vi "GetColoredBrush.vi"(0 "reference in":refnum<class "LcPictureBox.lvclass">, 1 "Alpha(100%)":dbl=100.0, 2 "Color(Black)":u32(colorbox), 3 "Pen(Width=1, Solid)":T1, 5 "Error In":errorcluster) -> (14 "reference out":refnum<class "LcPictureBox.lvclass">, 15 "SolidBrushRef":refnum<k24>, 19 "Error Out":errorcluster)   [LabVIEW 2020, in "LcPictureBox.lvclass"]
uses:
  LcPictureBox.lvclass
  Pen.ctl
  System.Drawing
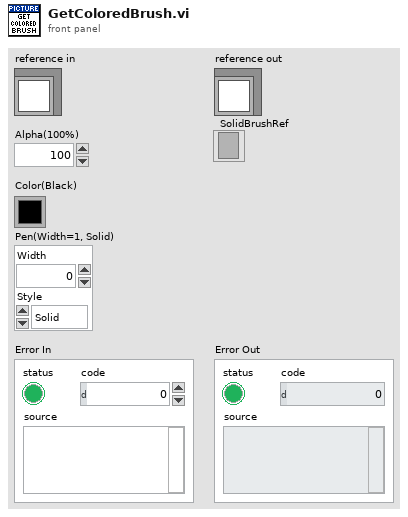
[diagram p1: front panel]
types:
  T1 = typedef "LcPictureBox.lvclass/Pen.ctl" = cluster{"Width":u16, "Style":enum32{"Solid", "Dash", "Dot", "DashDot", "DashDotDot"}}
  T2 = typedef "LcPictureBox.lvclass/ObjectAttributes.ctl" = cluster{"PictureBox":refnum<k24>, "ImageSize":cluster{"Width":i32, "Height":i32}, "PenMemory":map{cluster{"Alpha(100%)":dbl, "Color(Black)":u32, "Pen(Width=1, Solid)":T1}, refnum<k24>}, "GraphicsRef":refnum<k24>, "BrushMemory":map{cluster{"Alpha(100%)":dbl, "Color(Black)":u32}, refnum<k24>}, "Images":refnum<k24>[], "ImageIndex":i32, "BgColor(None)":u32, "LoadedImages":map{string, cluster{"ImageOut":refnum<k24>, "ImageSize":cluster{"Width":i32, "Height":i32}}}, "ColorsMemory":map{cluster{"Alpha(100%)":dbl, "Color(Black)":u32}, refnum<k24>}, "CacheSize":i32, "PictureBoxActiveXReference":refnum<vi>, "Scale":sgl, "Offset":cluster{"x":sgl, "y":sgl}, "zoom_center":cluster{"X":i32, "Y":i32}, "ImagesCreated":refnum<k24>[]}
  T3 = map{cluster{"Alpha(100%)":dbl, "Color(Black)":u32}, refnum<k24>}
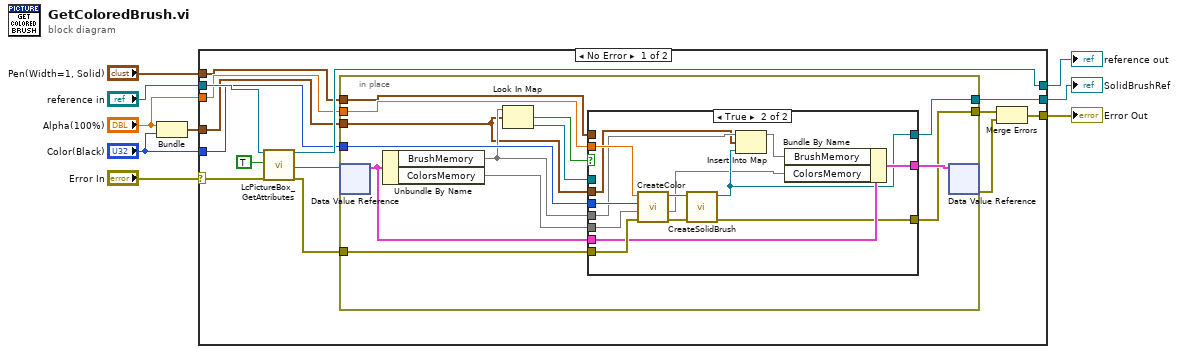
[diagram p0: block diagram]
diagram:
  n1 = Bundle("Alpha(100%)"="Alpha(100%)", "Color(Black)"="Color(Black)") -> (w5:cluster{"Alpha(100%)":dbl, "Color(Black)":u32})  [unwired: 1 in]
  n2 = case shown="No Error" "Error In" {
    selector: "Error In" -> [w22 w55]
    tunnel: [w19 w55] -> w8
    tunnel: [w20 w54] -> w6
    tunnel: "reference in" -> [w23 w54]
    tunnel: w5 -> [w16 _]
    tunnel: [w15 _] -> w4
    tunnel: "Alpha(100%)" -> [w14 _]
    tunnel: "Color(Black)" -> [w13 _]
    tunnel: "Pen(Width=1, Solid)" -> [w12 _]
    frame No Error {
      n3 = call "LcPictureBox_GetAttributes.vi"("reference in"=w23, "OnlyGetDvrReference(False)"=TRUE, "error in (no error)"=w22) -> ("reference out"=w20:refnum<class "LcPictureBox.lvclass">, "DataRef"=w18:refnum<data-value>, "error out"=w11:errorcluster)  [unwired: 13 in, 1 out]
      n4 = in-place {
        in-place-border: w16 -> [w25]
        in-place-border: [w32] -> w15
        in-place-border: w14 -> [w31]
        in-place-border: w13 -> [w30]
        in-place-border: w11 -> [w29]
        in-place-border: w12 -> [w28]
        in-place-border: [w27] -> w10
        n5 = in-place-dvr #1(w18) -> (w35:T2)  [unwired: 1 out]
        n6 = Unbundle By Name(w35) -> ("BrushMemory"=w26:T3, "ColorsMemory"=w24:T3)
        n7 = Look In Map(map=w26, key=w25) -> (key not found?=w34:bool, value=w33:refnum<k24>)  [unwired: 1 in]
        n8 = case shown="True" w34 {
          tunnel: [w37 w53] -> w36
          tunnel: w35 -> [w37 w48]
          tunnel: w33 -> [w39 _]
          tunnel: [w39 w43] -> w32
          tunnel: w31 -> [_ w52]
          tunnel: w30 -> [_ w51]
          tunnel: w29 -> [w38 w50]
          tunnel: w28 -> [_ _]
          tunnel: [w38 w40] -> w27
          tunnel: w26 -> [_ w47]
          tunnel: w25 -> [_ w45]
          tunnel: w24 -> [_ w42]
          frame False {
          }
          frame True {
            n9 = call "CreateColor.vi"("error in (no error)"=w50, "ColorsIn"=w42, "Color(Black)"=w51, "Alpha(100%)"=w52) -> ("error out"=w49:errorcluster, "ColorsOut"=w41:T3, "ColorRef"=w44:refnum<k24>)  [unwired: 5 in]
            n10 = call "CreateSolidBrush.vi"("error in (no error)"=w49, "ColorRef"=w44) -> ("error out"=w40:errorcluster, "SolidBrushRef"=w43:refnum<k24>)  [unwired: 8 in]
            n11 = Insert Into Map(map in=w47, key=w45, value=w43) -> (map out=w46:T3)  [unwired: 2 out]
            n12 = Bundle By Name(cluster=w48, "BrushMemory"=w46, "ColorsMemory"=w41) -> (w53:T2)
          }
        }
        n13 = in-place-dvr #1(w36) -> (w21:errorcluster)  [unwired: 1 out]
      }
      n14 = Merge Errors(w10, w21) -> (w19:errorcluster)
    }
    frame Error {
    }
  }
  "Error Out" <- w8
  "reference out" <- w6
  "SolidBrushRef" <- w4
